vi "Initialize.vi"(7 "Main VI":refnum<vi>, 8 "Error In":errorcluster, 9 "References":T1, 10 "Messages In":refnum<queue>, 11 "State In":T2) -> (0 "Error Out":errorcluster, 2 "Messages Out":refnum<queue>, 3 "State Out":T2)   [LabVIEW 2018, in "Bookmark Manager.lvlib"]
uses:
  Bookmark Manager.lvlib
  Controls/State.ctl
  <vilib>/addons/analyzer/_analyzerctrls.llb/VIAnCtl Analysis App Info.ctl
  Controls/Bookmark.ctl
  Controls/VI Identifier.ctl
  Controls/Bookmarks Groups.ctl
  Controls/Message.ctl
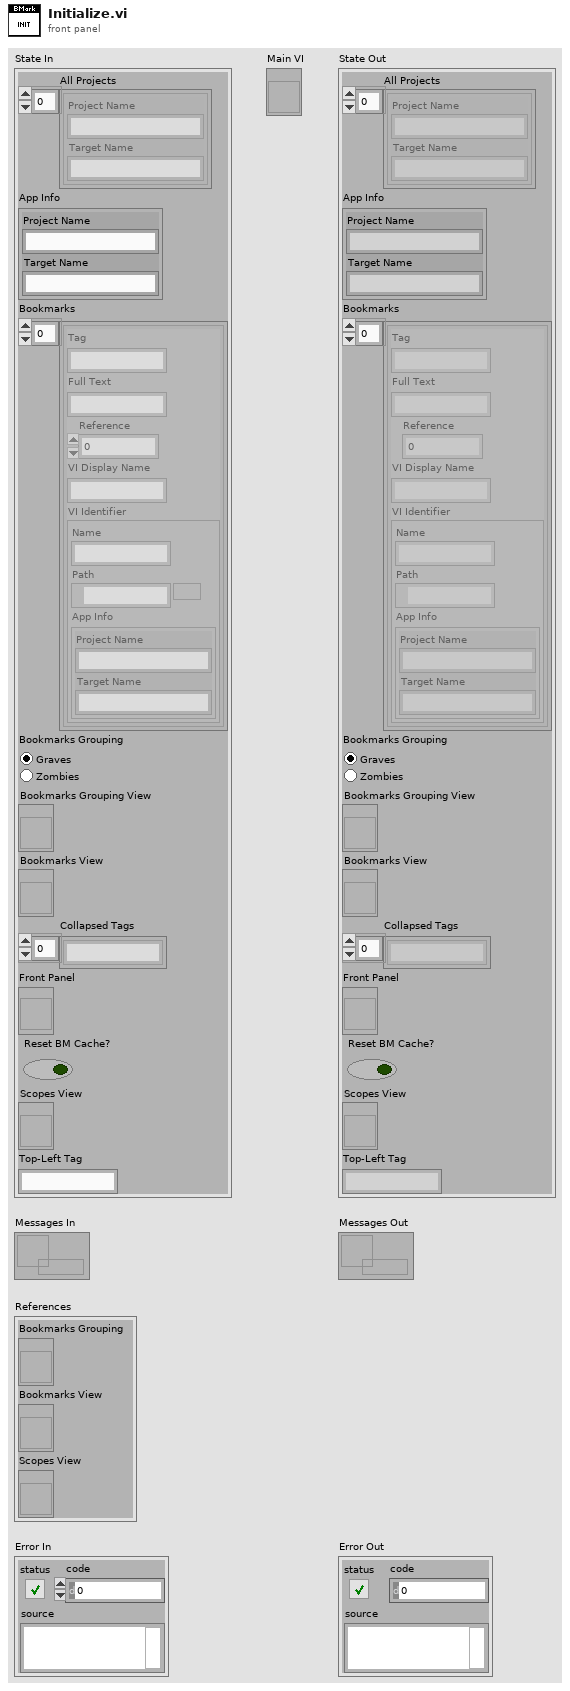
[diagram p1: front panel]
types:
  T1 = cluster{"Bookmarks Grouping":refnum<vi>, "Bookmarks View":refnum<vi>, "Scopes View":refnum<vi>}
  T2 = typedef "Bookmark Manager.lvlib/State.ctl" = cluster{"All Projects":T3[], "App Info":T3, "Bookmarks":T4[], "Bookmarks Grouping":T6, "Bookmarks Grouping View":refnum<vi>, "Bookmarks View":refnum<vi>, "Collapsed Tags":string[], "Front Panel":refnum<vi>, "Reset BM Cache?":bool, "Scopes View":refnum<vi>, "Top-Left Tag":string}
  T3 = typedef "VIAnCtl Analysis App Info.ctl" = cluster{"Project Name":string, "Target Name":string}
  T4 = typedef "Bookmark Manager.lvlib/Bookmark.ctl" = cluster{"Tag":string, "Full Text":string, "Reference":i32, "VI Display Name":string, "VI Identifier":T5}
  T5 = typedef "Bookmark Manager.lvlib/VI Identifier.ctl" = cluster{"Name":string, "Path":path, "App Info":T3}
  T6 = typedef "Bookmark Manager.lvlib/Bookmarks Groups.ctl" = enum32{"Graves", "Zombies"}
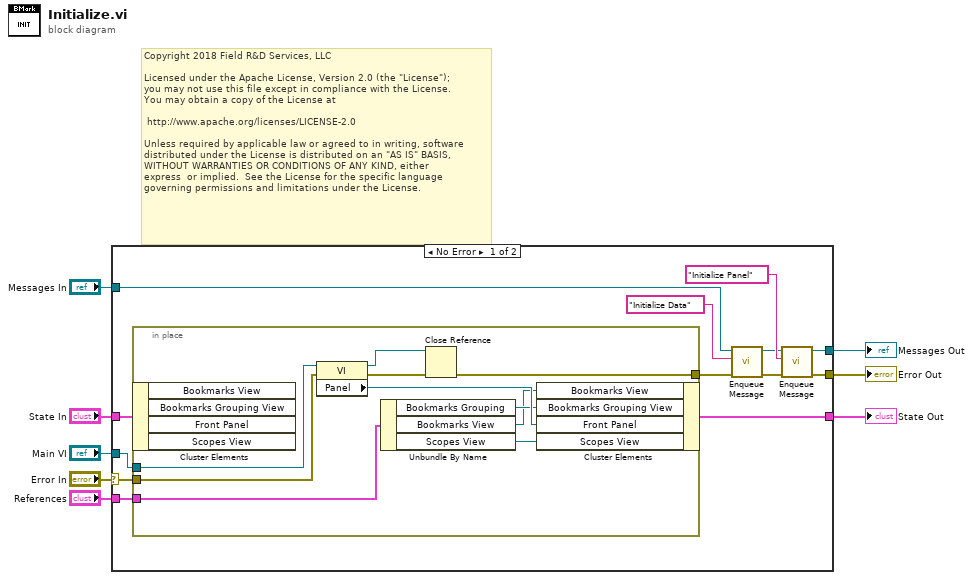
[diagram p0: block diagram]
diagram:
  # "Copyright 2018 Field R&D Services, LLC\n\nLicensed under the Apache License, Version 2.0 (the \"License\");\nyou may not use this file except in compliance with the License.\nYou may obtain a copy of the License at\n\n\thttp://www.apache.org/licenses/LICENSE-2.0\n\nUnless required by applicable law or agreed to in writing, software\ndistributed under the License is distributed on an \"AS IS\" BASIS,\nWITHOUT WARRANTIES OR CONDITIONS OF ANY KIND, either \nexpress  or implied.  See the License for the specific language \ngoverning permissions and limitations under the License."
  n1 = case shown="No Error" "Error In" {
    selector: "Error In" -> [w11 w34]
    tunnel: [w20 w34] -> w8
    tunnel: [w15 w33] -> w7
    tunnel: "State In" -> [w14 w33]
    tunnel: "Main VI" -> [w13 _]
    tunnel: "References" -> [w12 _]
    tunnel: "Messages In" -> [w10 w32]
    tunnel: [w9 w32] -> w1
    frame No Error {
      n2 = in-place {
        in-place-border: w11 -> [w27]
        in-place-border: [w29] -> w16
        in-place-border: w13 -> [w26]
        in-place-border: w12 -> [w25]
        n3 = in-place-cluster #1(w14) -> ()  [unwired: 4 out]
        n4 = property class="VI"(reference=w26, error in=w27) -> (reference out=w28:refnum<vi>, error out=w30:errorcluster, "Panel"=w31:refnum<vi>)
        n5 = Unbundle By Name(w25) -> ("Bookmarks Grouping"=w24:refnum<vi>, "Bookmarks View"=w23:refnum<vi>, "Scopes View"=w22:refnum<vi>)
        n6 = Close Reference(reference=w28, error in (no error)=w30) -> (error out=w29:errorcluster)
        n7 = in-place-cluster #1("Bookmarks View"=w23, "Bookmarks Grouping View"=w24, "Front Panel"=w31, "Scopes View"=w22) -> (w15:T2)
      }
      n8 = call "Enqueue Message.vi"("Error In"=w16, "Command"="Initialize Data", "Message Queue In"=w10) -> ("Error Out"=w19:errorcluster, "Message Queue Out"=w17:refnum<queue>)  [unwired: 7 in]
      n9 = call "Enqueue Message.vi"("Error In"=w19, "Command"="Initialize Panel", "Message Queue In"=w17) -> ("Error Out"=w20:errorcluster, "Message Queue Out"=w9:refnum<queue>)  [unwired: 7 in]
    }
    frame Error {
    }
  }
  "Error Out" <- w8
  "State Out" <- w7
  "Messages Out" <- w1
